vi "KE622x -- Execute Delta Meas.vi"(0 "Resource In":refnum<visa-resource-name>, 1 "Check For SCPI Errors? (T)":bool=TRUE, 5 "2812 -A Params In":T13={"Auto Range?"=FALSE, "Man / Selected\nRange"=enum."10mV", "Enable Digital\nFilter?"=FALSE, "Filter Type"=enum."Moving", "Filter Count"=10, "Filter\nWindow (%)"=0.01, "Enable Analog\nFilter?"=FALSE, "NPLCs"=5} {"Filter\nWindow (%)" min=0.0 max=10.0 step=0.01 format="%.2f"; "Filter Count" min=1 max=100; "NPLCs" min=1 max=10}, 7 "Delta Mode Params In":T2={"High Level (A)"=0.001, "Low Level (A)"=-0.001, "Delay (s)"=0.002, "Num Cycles Mode"=enum."Finite Count", "Finite Count"=10, "Abort On\nCompliance?"=FALSE, "Cold Swithing\nMode Enabled?"=FALSE} {"Finite Count" min=2 max=65536; "Low Level (A)" min=-0.105 max=0.0 format="%.3p"; "High Level (A)" min=0.0 max=0.105 format="%.3p"; "Delay (s)" min=0.001 max=9999.999 format="%.3f"}, 9 "Meas Units":T1=enum."Ohms", 11 "error in (no error)":errorcluster, 13 "Timeout (20000 ms)":u32=20000) -> (4 "Resource Out (dupl)":refnum<visa-resource-name>, 6 "2812 -A Params Out":T13={"Auto Range?"=FALSE, "Man / Selected\nRange"=enum."10mV", "Enable Digital\nFilter?"=FALSE, "Filter Type"=enum."Moving", "Filter Count"=10, "Filter\nWindow (%)"=0.01, "Enable Analog\nFilter?"=FALSE, "NPLCs"=5} {"Filter\nWindow (%)" min=0.0 max=10.0 step=0.01 format="%.2f"; "Filter Count" min=1 max=100; "NPLCs" min=1 max=60}, 8 "Delta Mode Params Out":T2={"High Level (A)"=0.001, "Low Level (A)"=-0.001, "Delay (s)"=0.002, "Num Cycles Mode"=enum."Finite Count", "Finite Count"=1, "Abort On\nCompliance?"=FALSE, "Cold Swithing\nMode Enabled?"=FALSE} {"Finite Count" min=1 max=65536; "Low Level (A)" min=-0.105 max=0.0 format="%.3p"; "High Level (A)" min=0.0 max=0.105 format="%.3p"; "Delay (s)" min=0.001 max=9999.999 format="%.3f"}, 10 "Timeout?":bool, 14 "Execution Time":dbl, 15 "error out":errorcluster)   [LabVIEW 2019, in "Keithley 622x.lvlib"]
doc: "Used to set up and execute a Delta Mode measurement. This VI accepts setup parameters for both the 2182/2182A and the 622x instruments."
uses:
  Keithley 622x.lvlib
  Configure/2182 -A/Low Level/Typedefs/KE2182 -- Voltage Ranges.ctl
  Configure/2182 -A/Low Level/Typedefs/KE2182 -- Filter Type.ctl
  Configure/2182 -A/Low Level/Typedefs/KE2182 -- Filter Count.ctl
  Configure/2182 -A/Low Level/Typedefs/KE2182 -- Filter Window.ctl
  Configure/2182 -A/Low Level/Typedefs/KE2182 -- NPLCs.ctl
  Configure/Delta PDelta DCon Modes/Typedefs/KE622x -- Delta Mode Params.ctl
  Configure/Delta PDelta DCon Modes/Low Level/Typedefs/KE622x -- Delta PDelta Mode High Level.ctl
  Configure/Delta PDelta DCon Modes/Low Level/Typedefs/KE622x -- Delta PDelta Mode Low Level.ctl
  Configure/Delta PDelta DCon Modes/Low Level/Typedefs/KE622x -- Delta DCon Mode Delay.ctl
  Configure/Delta PDelta DCon Modes/Low Level/Typedefs/KE622x -- Delta PDelta Mode Num Cycles Mode.ctl
  Configure/Delta PDelta DCon Modes/Low Level/Typedefs/KE622x -- Delta PDelta Mode Num Cycles.ctl
  Configure/Units/Typedefs/KE622x -- Voltage Meas Units.ctl
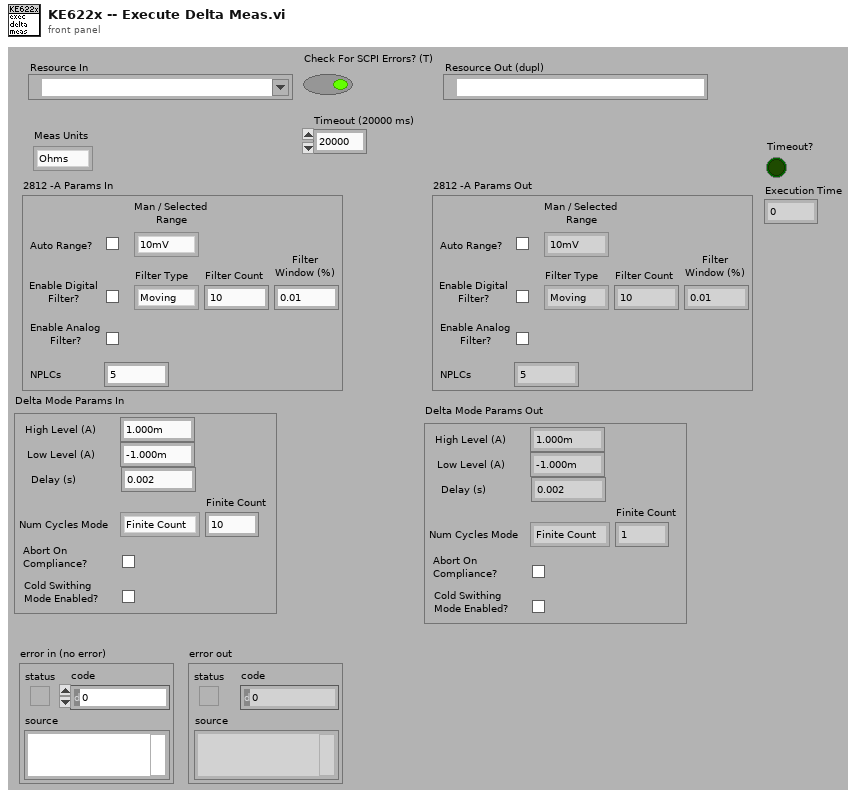
[diagram p1: front panel]
types:
  T1 = typedef "Keithley 622x.lvlib/KE622x -- Voltage Meas Units.ctl" = enum16{"Volts", "Ohms", "Watts", "Siemens"}
  T2 = typedef "Keithley 622x.lvlib/KE622x -- Delta Mode Params.ctl" = cluster{"High Level (A)":T3, "Low Level (A)":T4, "Delay (s)":T5, "Num Cycles Mode":T6, "Finite Count":T7, "Abort On\nCompliance?":bool, "Cold Swithing\nMode Enabled?":bool}
  T3 = typedef "Keithley 622x.lvlib/KE622x -- Delta PDelta Mode High Level.ctl" = dbl
  T4 = typedef "Keithley 622x.lvlib/KE622x -- Delta PDelta Mode Low Level.ctl" = dbl
  T5 = typedef "Keithley 622x.lvlib/KE622x -- Delta DCon Mode Delay.ctl" = dbl
  T6 = typedef "Keithley 622x.lvlib/KE622x -- Delta PDelta Mode Num Cycles Mode.ctl" = enum16{"Finite Count", "Infinite"}
  T7 = typedef "Keithley 622x.lvlib/KE622x -- Delta PDelta Mode Num Cycles.ctl" = u32
  T8 = typedef "Keithley 622x.lvlib/KE2182 -- Voltage Ranges.ctl" = enum16{"10mV", "100mV", "1V", "10V", "100V"}
  T9 = typedef "Keithley 622x.lvlib/KE2182 -- Filter Type.ctl" = enum16{"Moving", "Repeat"}
  T10 = typedef "Keithley 622x.lvlib/KE2182 -- Filter Count.ctl" = u32
  T11 = typedef "Keithley 622x.lvlib/KE2182 -- Filter Window.ctl" = dbl
  T12 = typedef "Keithley 622x.lvlib/KE2182 -- NPLCs.ctl" = u32
  T13 = cluster{"Auto Range?":bool, "Man / Selected\nRange":T8, "Enable Digital\nFilter?":bool, "Filter Type":T9, "Filter Count":T10, "Filter\nWindow (%)":T11, "Enable Analog\nFilter?":bool, "NPLCs":T12}
  T14 = typedef "Keithley 622x.lvlib/KE622x -- Meas Event Reg State.ctl" = cluster{"B0, ROF:  KE2182A Delta Reading Overflow Event?":bool, "B1, Int:  Interlock OK Event?":bool, "B2, Temp:  Over Temperature Event?":bool, "B3, Comp:  Compliance Event?":bool, "B5, RAV:  Delta Reading Available Event?":bool, "B6, TN:  User Defined Reading Number Stored In Buffer Event?":bool, "B7, BAV:  At Least 2 Readings Stored In Buffer Event?":bool, "B12, BQF:  Buffer Quarter Full Event?":bool, "B8, BHF:  Buffer Half Full Event?":bool, "B13, B3QF:  Buffer 3/4 Full Event?":bool, "B9, BFL:  Buffer Full Event?":bool}
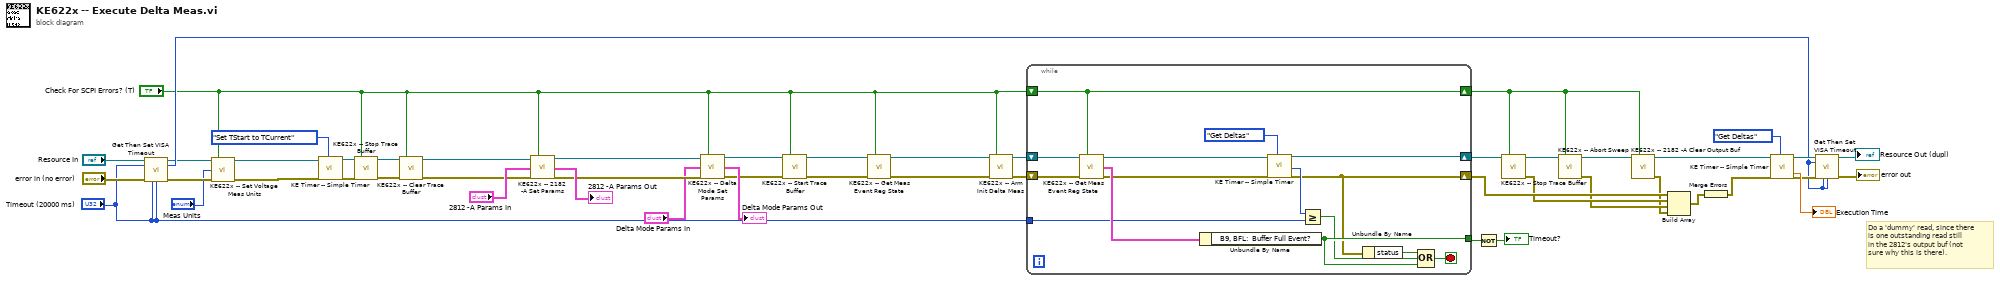
[diagram p0: block diagram]
diagram:
  # "Do a 'dummy' read, since there\nis one outstanding read still\nin the 2812's output buf (not\nsure why this is there)."
  n1 = call "Get Then Set VISA Timeout.vi"("VISA Resource Name In"="Resource In", "New Timeout (msecs)"="Timeout (20000 ms)", "error in (no error)"="error in (no error)", "Max Timeout (300 secs)"="Timeout (20000 ms)", "Min Timeout (3 secs)"="Timeout (20000 ms)") -> ("VISA Resource Name Out (dupl)"=w6:refnum<visa-resource-name>, "Old Timeout (msecs)"=w7:u32, "error out"=w5:errorcluster)  [unwired: 7 in, 1 out]
  n2 = call "KE622x -- Set Voltage Meas Units.vi"("Resource In"=w6, "Check For SCPI Errors? (T)"="Check For SCPI Errors? (T)", "Voltage Meas Units"="Meas Units", "error in (no error)"=w5) -> ("Resource Out (dupl)"=w2:refnum<visa-resource-name>, "error out"=w4:errorcluster)  [unwired: 10 in]
  n3 = call "KE Timer -- Simple Timer.vi"("Resource In"=w2, "error in (no error)"=w4, "Action"=enum16{"Set TStart to TCurrent", "Get Deltas"}."Set TStart to TCurrent") -> ("Resource Out (dupl)"=w26:refnum<visa-resource-name>, "error out (dupl)"=w25:errorcluster)  [unwired: 7 in, 8 out]
  n4 = call "KE622x -- Stop Trace Buffer.vi"("Resource In"=w26, "Check For SCPI Errors? (T)"="Check For SCPI Errors? (T)", "error in (no error)"=w25) -> ("Resource Out (dupl)"=w44:refnum<visa-resource-name>, "error out"=w43:errorcluster)  [unwired: 11 in]
  n5 = call "KE622x -- Clear Trace Buffer.vi"("Resource In"=w44, "Check For SCPI Errors? (T)"="Check For SCPI Errors? (T)", "error in (no error)"=w43) -> ("Resource Out (dupl)"=w22:refnum<visa-resource-name>, "error out"=w21:errorcluster)  [unwired: 11 in]
  n6 = call "KE622x -- 2182 -A Set Params.vi"("622x Resource In"=w22, "Check For SCPI Errors? (T)"="Check For SCPI Errors? (T)", "2812 -A Params In"="2812 -A Params In", "error in (no error)"=w21) -> ("622x Resource Out (dupl)"=w48:refnum<visa-resource-name>, "2812 -A Params Out"=→"2812 -A Params Out":T13, "error out"=w47:errorcluster)  [unwired: 9 in]
  n7 = call "KE622x -- Delta Mode Set Params.vi"("Resource In"=w48, "Check For SCPI Errors? (T)"="Check For SCPI Errors? (T)", "Delta Mode Params In"="Delta Mode Params In", "error in (no error)"=w47) -> ("Resource Out (dupl)"=w42:refnum<visa-resource-name>, "Delta Mode Params Out"=→"Delta Mode Params Out":T2, "error out"=w41:errorcluster)  [unwired: 9 in]
  n8 = call "KE622x -- Start Trace Buffer.vi"("Resource In"=w42, "Check For SCPI Errors? (T)"="Check For SCPI Errors? (T)", "error in (no error)"=w41) -> ("Resource Out (dupl)"=w39:refnum<visa-resource-name>, "error out"=w40:errorcluster)  [unwired: 11 in]
  n9 = call "KE622x -- Get Meas Event Reg State.vi"("VISA Resource In"=w39, "Error Query (T)?"="Check For SCPI Errors? (T)", "error in (no error)"=w40) -> ("VISA Resource Out (dupl)"=w24:refnum<visa-resource-name>, "error out"=w23:errorcluster)  [unwired: 10 in, 1 out]
  n10 = call "KE622x -- Arm Init Delta Meas.vi"("Resource In"=w24, "Check For SCPI Errors? (T)"="Check For SCPI Errors? (T)", "error in (no error)"=w23) -> ("Resource Out (dupl)"=w36:refnum<visa-resource-name>, "error out"=w37:errorcluster)  [unwired: 11 in]
  n11 = while {
    shift-right: [w53] -> w19
    shift-left: w37 -> [w65]
    shift-right: [w55] -> w33
    shift-left: w36 -> [w64]
    tunnel: [w57] -> w35
    shift-right: [w54] -> w30
    shift-left: "Check For SCPI Errors? (T)" -> [w54]
    tunnel: "Timeout (20000 ms)" -> [w51]
    stop <- w58 stop-if-true
    n12 = call "KE622x -- Get Meas Event Reg State.vi"("VISA Resource In"=w64, "Error Query (T)?"=w54, "error in (no error)"=w65) -> ("VISA Resource Out (dupl)"=w61:refnum<visa-resource-name>, "KE622x Meas Event Reg"=w63:T14, "error out"=w62:errorcluster)  [unwired: 10 in]
    n13 = Unbundle By Name(w63) -> ("B9, BFL:  Buffer Full Event?"=w57:bool)
    n14 = call "KE Timer -- Simple Timer.vi"("Resource In"=w61, "error in (no error)"=w62, "Action"=enum16{"Set TStart to TCurrent", "Get Deltas"}."Get Deltas") -> ("Resource Out (dupl)"=w55:refnum<visa-resource-name>, "TCurrent - TStart (ms)"=w59:u32, "error out (dupl)"=w53:errorcluster)  [unwired: 7 in, 7 out]
    n15 = Greater Or Equal?(x=w59, y=w51) -> (x >= y?=w56:bool)
    n16 = Unbundle By Name(w53) -> ("status"=w52:bool)
    n17 = Compound Arithmetic op=OR(w52, w56, w57) -> (w58:bool)
  }
  n18 = Not(x=w35) -> (.not. x?=→"Timeout?":bool)
  n19 = call "KE622x -- Stop Trace Buffer.vi"("Resource In"=w33, "Check For SCPI Errors? (T)"=w30) -> ("Resource Out (dupl)"=w32:refnum<visa-resource-name>, "error out"=w18:errorcluster)  [unwired: 12 in]
  n20 = call "KE622x -- Abort Sweep.vi"("Resource In"=w32, "Check For SCPI Errors? (T)"=w30) -> ("Resource Out (dupl)"=w31:refnum<visa-resource-name>, "error out"=w17:errorcluster)  [unwired: 12 in]
  n21 = call "KE622x -- 2182 -A Clear Output Buf.vi"("622x Resource In"=w31, "Check For SCPI Errors? (T)"=w30) -> ("622x Resource Out (dupl)"=w29:refnum<visa-resource-name>, "error out"=w16:errorcluster)  [unwired: 11 in, 1 out]
  n22 = Build Array(w19, w18, w17, w16) -> (w20:errorcluster[])
  n23 = Merge Errors(w20) -> (w15:errorcluster)
  n24 = call "KE Timer -- Simple Timer.vi"("Resource In"=w29, "error in (no error)"=w15, "Action"=enum16{"Set TStart to TCurrent", "Get Deltas"}."Get Deltas") -> ("TCurrent - TStart (s)"=→"Execution Time":dbl, "Resource Out (dupl)"=w8:refnum<visa-resource-name>, "error out (dupl)"=w11:errorcluster)  [unwired: 7 in, 7 out]
  n25 = call "Get Then Set VISA Timeout.vi"("VISA Resource Name In"=w8, "New Timeout (msecs)"=w7, "error in (no error)"=w11, "Max Timeout (300 secs)"=w7, "Min Timeout (3 secs)"=w7) -> ("VISA Resource Name Out (dupl)"=→"Resource Out (dupl)":refnum<visa-resource-name>, "error out"=→"error out":errorcluster)  [unwired: 7 in, 2 out]
